vi "EnableCache x86.vi"(8 "error in (no error)":errorcluster) -> (0 "error out":errorcluster)   [LabVIEW 2014]
uses:
  Invalidate_Cache.dll
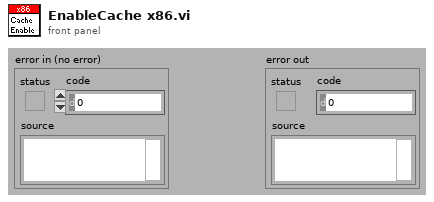
[diagram p1: front panel]
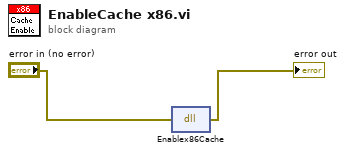
[diagram p0: block diagram]
diagram:
  n1 = dll-call lib="C:/Users/nitest/Documents/GitHub/IntegrationTesting/RT-Cert/tests_auto/performance/CommonSubVIs/Cache/Invalidate_Cache.dll" fn="Enablex86Cache" ("vxWorks:cacheInvalidate")(error in="error in (no error)") -> (error out=→"error out":errorcluster)  [unwired: 3 in, 1 out]
